vi "TDS Make Connection.vi"(8 "error in (no error)":errorcluster, 9 "State":bool, 10 "Connection Configuration":string, 11 "Address":string) -> (0 "error out":errorcluster)   [LabVIEW 2025, in "Interface Functions.lvlib"]
uses:
  Interface Functions.lvlib
  <vilib>/Utility/error.llb/Trim Whitespace One-Sided.vi
panel:
  # "Make Connection"
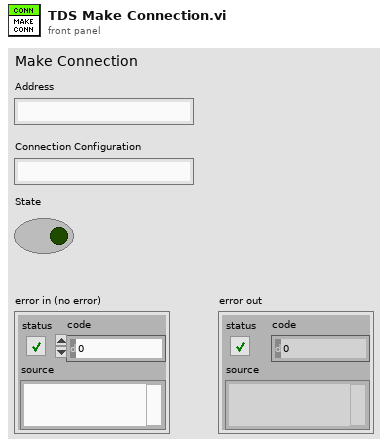
[diagram p1: front panel]
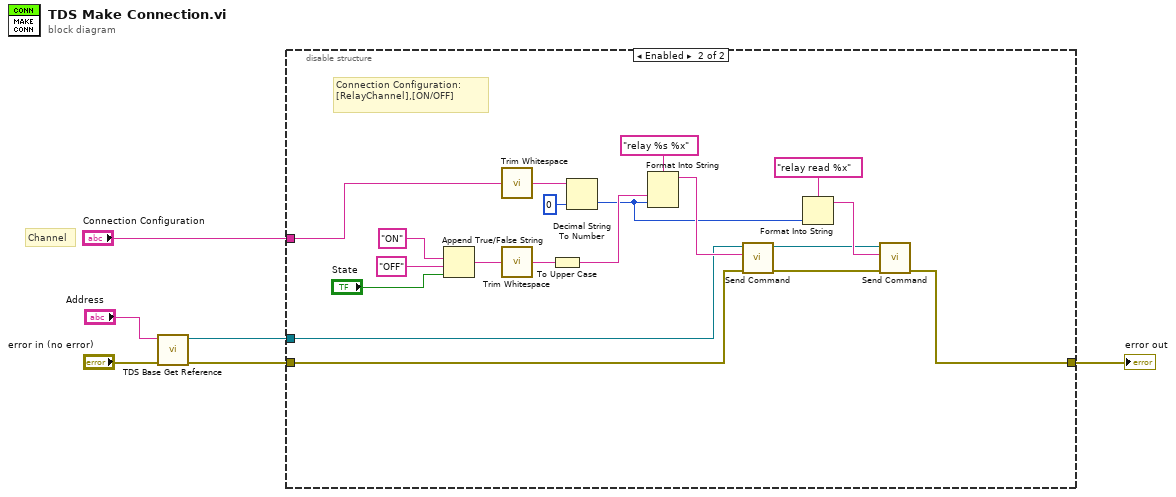
[diagram p0: block diagram]
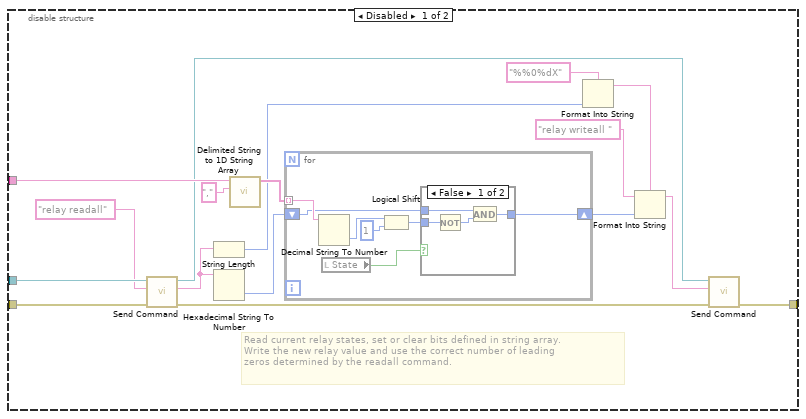
[diagram p2: hidden frame]
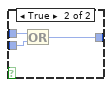
[diagram p3: hidden frame]
diagram:
  # "Channel"
  n1 = call "TDS Base Get Reference.vi"("error in (no error)"="error in (no error)", "Address"="Address") -> ("error out"=w3:errorcluster, "Reference"=w4:refnum<visa-resource-name>)  [unwired: 8 in]
  n2 = disable-structure shown="Enabled" {
    disable-tunnel: w4 -> [w23 w48]
    disable-tunnel: w3 -> [w22 w51]
    disable-tunnel: "Connection Configuration" -> [w21 w41]
    disable-tunnel: [w7 w46] -> w1
    frame Disabled {
      # "Read current relay states, set or clear bits defined in string array.\nWrite the new relay value and use the correct number of leading \nzeros determined by the readall command."
      n3 = call "Send Command.vi"("error in (no error)"=w22, "Command"="relay readall", "VISA resource name"=w23) -> ("error out"=w10:errorcluster, "Read Value"=w12:string, "VISA resource name out"=w9:refnum<visa-resource-name>)  [unwired: 6 in]
      n4 = String Length(string=w12) -> (length=w14:i32)
      n5 = Hexadecimal String To Number(string=w12) -> (number=w11:u32)  [unwired: 2 in, 1 out]
      n6 = call <vilib>:"Delimited String to 1D String Array.vi"("delimiter"="," ("delimiter (Tab)"), "delimited string"=w21) -> ("string array"=w18:string[])  [unwired: 9 in]
      n7 = for {
        tunnel: w18 -> [w29] mode=indexing
        shift-right: [w26] -> w15
        shift-left: w11 -> [w25]
        n8 = Decimal String To Number(string=w29) -> (number=w28:i32)  [unwired: 2 in, 1 out]
        n9 = local read "State"() -> (w24:bool)
        n10 = Logical Shift(y=w28, x=u32 1) -> (x << y=w27:u32)
        n11 = case shown="False" w24 {
          tunnel: w27 -> [w34 w37]
          tunnel: [w31 w36] -> w26
          tunnel: w25 -> [w32 w35]
          frame False {
            n12 = Not(x=w34) -> (.not. x?=w33:u32)
            n13 = And(x=w32, y=w33) -> (x .and. y?=w31:u32)
          }
          frame True {
            n14 = Or(x=w35, y=w37) -> (x .or. y?=w36:u32)
          }
        }
      }
      n15 = Format Into String(format string="%%0%dX" ("write buffer"), w14) -> (resulting string=w16:string)  [unwired: 2 in, 1 out]
      n16 = Format Into String(format string=w16, initial string="relay writeall ", w15) -> (resulting string=w8:string)  [unwired: 1 in, 1 out]
      n17 = call "Send Command.vi"("error in (no error)"=w10, "Command"=w8, "VISA resource name"=w9) -> ("error out"=w7:errorcluster)  [unwired: 6 in, 2 out]
    }
    frame Enabled {
      # "Connection Configuration:\n[RelayChannel],[ON/OFF]"
      n18 = Append True/False String(1:"State", 2:"OFF" ("false string"), 3:"ON" ("true string")) -> (0:w40:string)  [unwired: 1 in]
      n19 = call <vilib>:"Trim Whitespace.vi"("string"=w41) -> ("trimmed string"=w54:string)  [unwired: 1 in]
      n20 = call <vilib>:"Trim Whitespace.vi"("string"=w40) -> ("trimmed string"=w55:string)  [unwired: 1 in]
      n21 = To Upper Case(1:w55) -> (0:w53:string)
      n22 = Decimal String To Number(string=w54, default (0L)=u32 0) -> (number=w50:u32)  [unwired: 1 in, 1 out]
      n23 = Format Into String(format string="relay %s %x" ("write buffer"), w53, w50) -> (resulting string=w52:string)  [unwired: 2 in, 1 out]
      n24 = call "Send Command.vi"("error in (no error)"=w51, "Command"=w52, "VISA resource name"=w48) -> ("error out"=w49:errorcluster, "VISA resource name out"=w45:refnum<visa-resource-name>)  [unwired: 6 in, 1 out]
      n25 = Format Into String(format string="relay read %x" ("write buffer"), w50) -> (resulting string=w47:string)  [unwired: 2 in, 1 out]
      n26 = call "Send Command.vi"("error in (no error)"=w49, "Command"=w47, "VISA resource name"=w45) -> ("error out"=w46:errorcluster)  [unwired: 6 in, 2 out]
    }
  }
  "error out" <- w1
